vi "Designing Message Loop.vi"(8 "error in (no error)":errorcluster, 9 "Data Queue":refnum<queue>, 10 "Data Notifier":refnum<notifier>, 11 "Message Queues":T1) -> (0 "error out":errorcluster)   [LabVIEW 2025]
uses:
  support/Message Queue/All Message Queues.ctl
  support/Message Queue/Message Cluster.ctl
  controls/Tuners.ctl
  controls/Constants.ctl
  Designing Loop Enum.ctl
  <vilib>/Utility/error.llb/Error Cluster From Error Code.vi
  <vilib>/ErrorRing/Error Ring.xnode
  support/Message Queue/Message Queue.lvlib
  Results.ctl
panel:
  # "Simulator Fit"
  # "Empirical Fit"
  # "="
  # "P"
  # "* X"
  # "P"
  # "="
  # "* X"
  # "drop"
  # "drop"
  # "Simulator Fit"
  # "Empirical Fit"
  # "="
  # "P"
  # "* X"
  # "P"
  # "="
  # "* X"
  # "drop"
  # "drop"
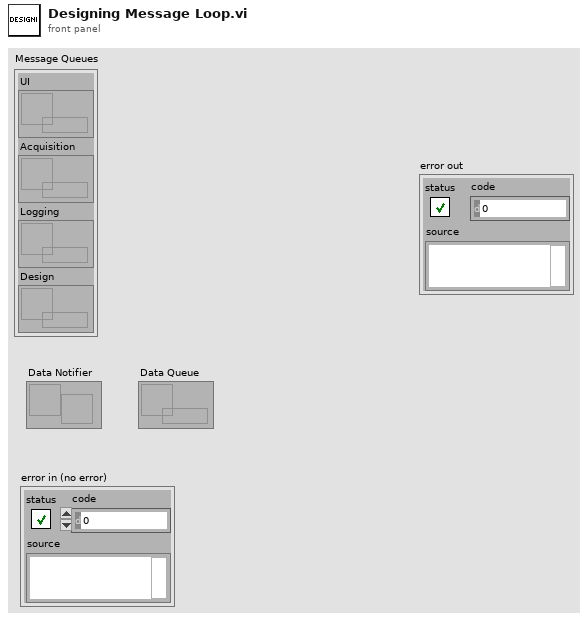
[diagram p1: front panel]
types:
  T1 = typedef "Message Queue.lvlib/All Message Queues.ctl" = cluster{"UI":refnum<queue>, "Acquisition":refnum<queue>, "Logging":refnum<queue>, "Design":refnum<queue>}
  T2 = typedef "Designing Loop Enum.ctl" = enum16{"Output New Results", "Start"}
  T3 = typedef "Results.ctl" = cluster{"Waveform":waveform(dbl), "Design Results":cluster{"Model Validation: Simulated vs. Empirical Airflow Data":cluster{dbl[], dbl[]}[], "Amplitude - Empirical":string, "Power - Empirical":string, "Amplitude - Sim":string, "Power - Sim":string, "Flow Type":u32, "Optimized Inlet \nOrifice Diameter (in)":dbl, "Flow Type Name":string}}
  T4 = typedef "Constants.ctl" = cluster{"P_amb (psia)":dbl, "T_in (Deg F)":dbl, "R_air (ft*lbf)/(lbm*R)":dbl, "g_c (lbm*ft)/(lbf*s^2)":dbl, "specific heat ratio":dbl, "Viscousity (lbm)/(ft*s)":dbl, "Cd":dbl, "Mass Flow (lbm/min) vs. Pressure Drop (inH2O) - Real Data":dbl[][]}
  T5 = typedef "Tuners.ctl" = cluster{"Inlet Diameter (in)":dbl, "Outlet Diameter (in)":dbl, " Length (in)":dbl, "   Diameter (in)":dbl, "D_h (in)":dbl, "OAR":dbl, "Run Optimizer":bool}
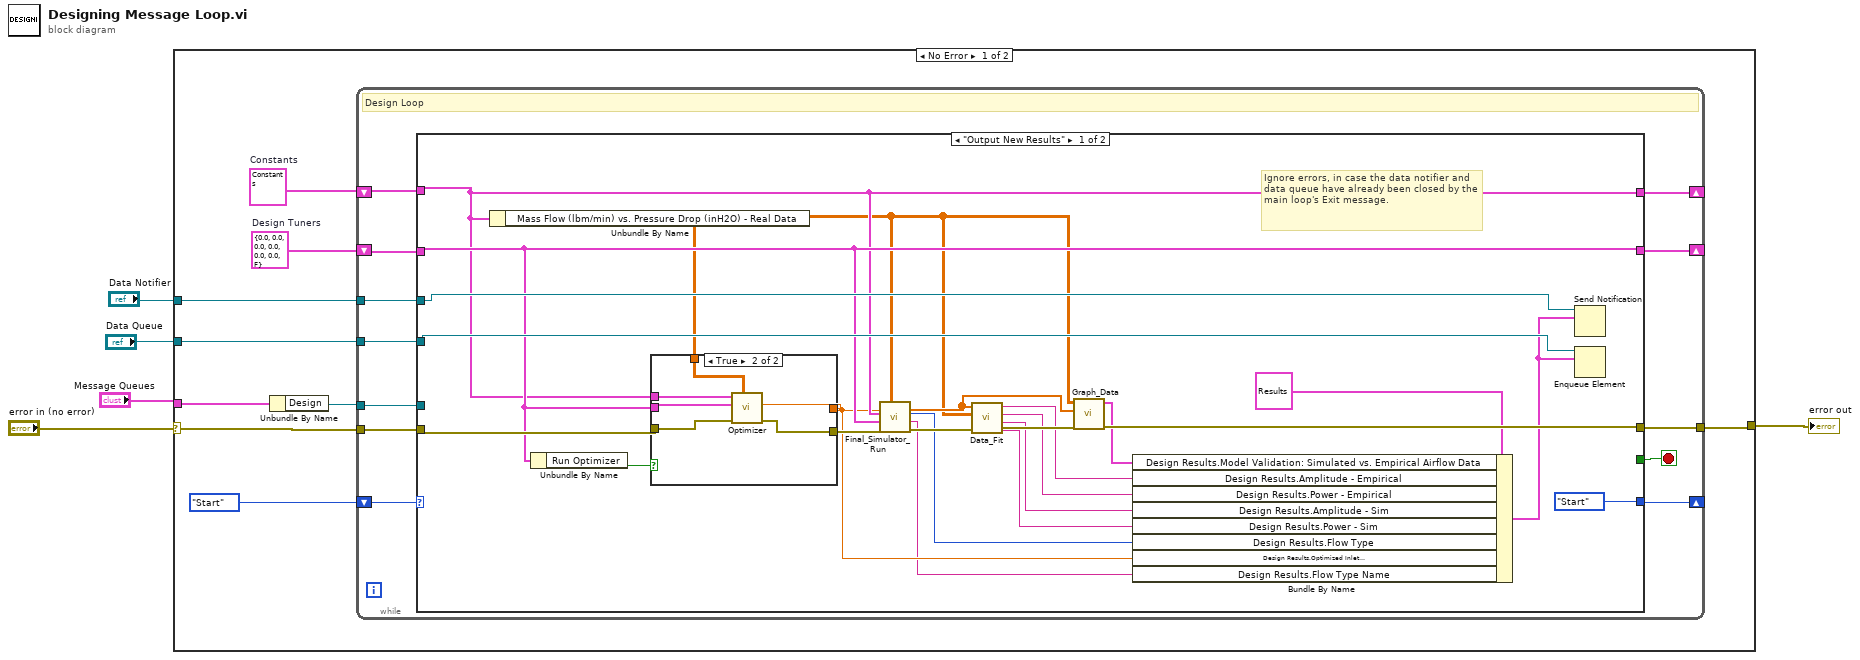
[diagram p0: block diagram]
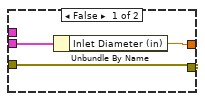
[diagram p2: hidden frame]
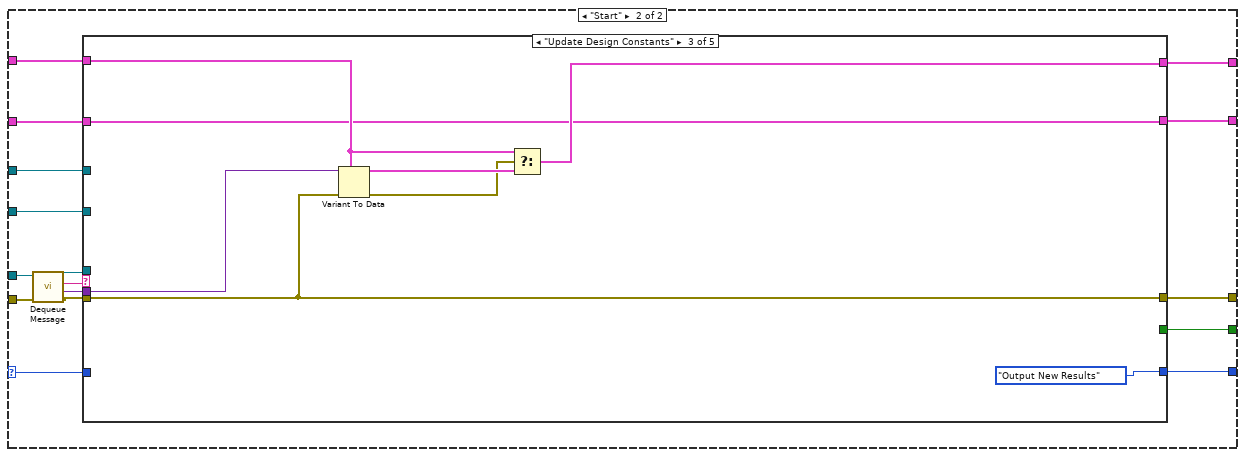
[diagram p3: hidden frame]
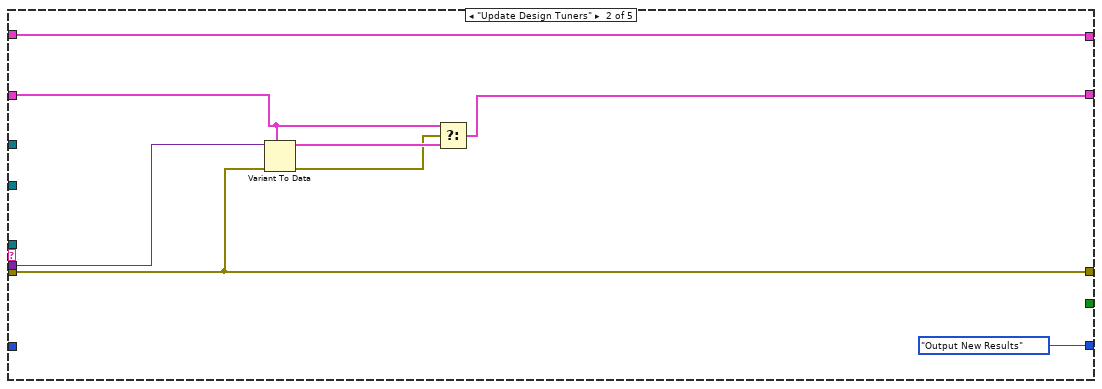
[diagram p5: hidden frame]
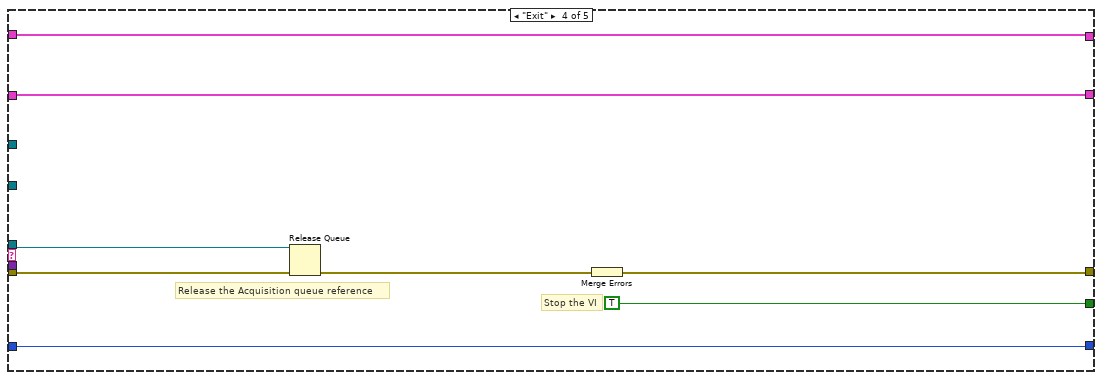
[diagram p6: hidden frame]
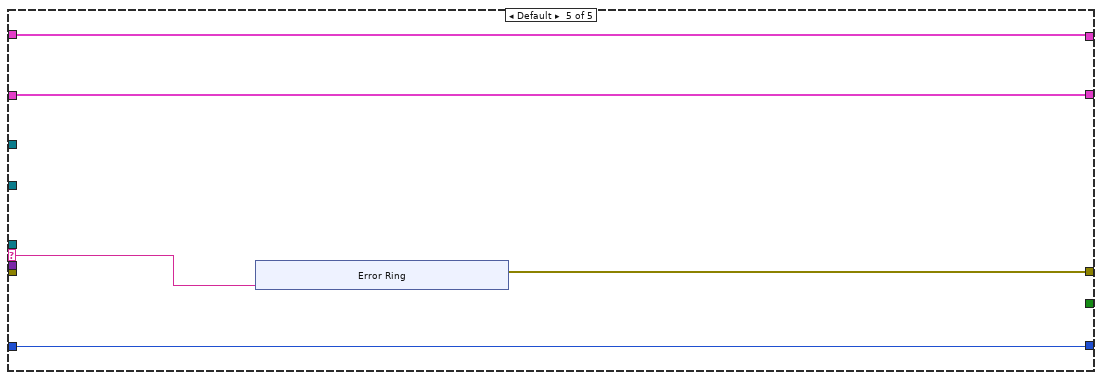
[diagram p7: hidden frame]
diagram:
  n1 = case shown="No Error" "error in (no error)" {
    selector: "error in (no error)" -> [w12 w115]
    tunnel: "Message Queues" -> [w14 _]
    tunnel: [w11 w115] -> w3
    tunnel: "Data Notifier" -> [w8 _]
    tunnel: "Data Queue" -> [w7 _]
    frame No Error {
      w9 = T4 {"P_amb (psia)"=14.7, "T_in (Deg F)"=530.0, "R_air (ft*lbf)/(lbm*R)"=53.35, "g_c (lbm*ft)/(lbf*s^2)"=32.17, "specific heat ratio"=1.4, "Viscousity (lbm)/(ft*s)"=1.21e-05, "Cd"=0.61, "Mass Flow (lbm/min) vs. Pressure Drop (inH2O) - Real Data"=[[0.5, 0.015], [1.0, 0.062], [1.5, 0.141], [2.0, 0.252], [2.5, 0.395], [3.5, 0.778]]}  # Constants
      w10 = T5 {"Inlet Diameter (in)"=0.0, "Outlet Diameter (in)"=0.0, " Length (in)"=0.0, "   Diameter (in)"=0.0, "D_h (in)"=0.0, "OAR"=0.0, "Run Optimizer"=FALSE}  # Design Tuners
      n2 = Unbundle By Name(w14) -> ("Design"=w13:refnum<queue>)
      n3 = while {
        tunnel: w13 -> [w26]
        tunnel: w12 -> [w25]
        tunnel: [w24] -> w11
        shift-right: [w22] -> _
        shift-left: w10 -> [w23]
        shift-right: [w20] -> _
        shift-left: w9 -> [w21]
        tunnel: w8 -> [w18]
        tunnel: w7 -> [w17]
        shift-right: [w15] -> _
        shift-left: Designing_Loop_Enum."Start" -> [w16]
        stop <- w19 stop-if-true
        # "Design Loop"
        n4 = case shown="\"Output New Results\"" w16 {
          selector: w16 -> [_ w59]
          tunnel: w26 -> [_ w74]
          tunnel: w25 -> [w42 w72]
          tunnel: [w41 w71] -> w24
          tunnel: w23 -> [w39 w69]
          tunnel: [w39 w68] -> w22
          tunnel: w21 -> [w38 w66]
          tunnel: [w38 w65] -> w20
          tunnel: [_ w64] -> w19
          tunnel: w18 -> [w44 w62]
          tunnel: w17 -> [w43 w61]
          tunnel: [Designing_Loop_Enum."Start" w60] -> w15
          frame "Output New Results" {
            # "Ignore errors, in case the data notifier and data queue have already been closed by the main loop's Exit message."
            n5 = Unbundle By Name(w38) -> ("Mass Flow (lbm/min) vs. Pressure Drop (inH2O) - Real Data"=w37:dbl[][])
            n6 = Unbundle By Name(w39) -> ("Run Optimizer"=w45:bool)
            n7 = case shown="True" w45 {
              tunnel: [w52 w54] -> w46
              tunnel: [w50 w58] -> w29
              tunnel: w42 -> [w52 w57]
              tunnel: w39 -> [w51 w55]
              tunnel: w37 -> [_ w56]
              tunnel: w38 -> [_ w53]
              frame False {
                n8 = Unbundle By Name(w51) -> ("Inlet Diameter (in)"=w50:dbl)
              }
              frame True {
                n9 = call "Optimizer.vi"("Mass Flow (lbm/min) vs. Pressure Drop (inH2O) - Real Data"=w56, "error in"=w57, "Tuners"=w55, "System Configuration"=w53) -> ("error out"=w54:errorcluster, "optimized_diameter"=w58:dbl)  [unwired: 6 in]
              }
            }
            n10 = call "Final_Simulator_Run.vi"("Mass Flow (lbm/min) vs. Pressure Drop (inH2O) - Real Data"=w37, "error in (no error)"=w46, "Tuners"=w39, "System Configuration"=w38, "d_in_guess"=w29) -> ("error out"=w48:errorcluster, "Flow Type Name"=w28:string, "Flow Type"=w30:u32, "total_dp_inh2o"=w47:dbl[])  [unwired: 3 in]
            n11 = call "Data_Fit.vi"("error in (no error)"=w48, "Mass Flow (lbm/min) vs. Pressure Drop (inH2O) - Real Data"=w37, "total_dp_inh2o"=w47) -> ("Power - Sim"=w31:string, "Amplitude - Sim"=w32:string, "Power - Empirical"=w33:string, "Amplitude - Empirical"=w34:string, "error out"=w49:errorcluster)  [unwired: 4 in]
            n12 = call "Graph_Data.vi"("error in (no error)"=w49, "total_dp_inh2o"=w47, "Mass Flow (lbm/min) vs. Pressure Drop (inH2O) - Real Data"=w37) -> ("error out"=w41:errorcluster, "Model Validation"=w35:cluster{dbl[], dbl[]}[])  [unwired: 7 in]
            n13 = Bundle By Name(cluster=T3 {"Waveform"={"t0"=timestamp(0 s since 1904-01-01), "dt"=1.0, "Y"=[]}, "Design Results"={"Model Validation: Simulated vs. Empirical Airflow Data"=[], "Amplitude - Empirical"="", "Power - Empirical"="", "Amplitude - Sim"="", "Power - Sim"="", "Flow Type"=0, "Optimized Inlet \nOrifice Diameter (in)"=0.0, "Flow Type Name"=""}} ("Results 2"), "Design Results.Model Validation: Simulated vs. Empirical Airflow Data"=w35, "Design Results.Amplitude - Empirical"=w34, "Design Results.Power - Empirical"=w33, "Design Results.Amplitude - Sim"=w32, "Design Results.Power - Sim"=w31, "Design Results.Flow Type"=w30, "Design Results.Optimized Inlet \nOrifice Diameter (in)"=w29, "Design Results.Flow Type Name"=w28) -> (w27:T3)
            n14 = Send Notification(notification=w27, notifier=w44) -> ()  [unwired: 1 in, 2 out]
            n15 = Enqueue Element(queue=w43, element=w27) -> ()  [unwired: 2 in, 3 out]
          }
          frame "Start" {
            n16 = call "Dequeue Message.vi"("error in (no error)"=w72, "Message Queue"=w74) -> ("error out"=w70:errorcluster, "Message Data"=w67:variant, "Message"=w73:string, "dup Message Queue"=w63:refnum<queue>)  [unwired: 6 in]
            n17 = case shown="\"Update Design Constants\"" w73 {
              selector: w73 -> [_ _ _ _ w107]
              tunnel: [w78 w83 w92 w99 w106] -> w71
              tunnel: w70 -> [w78 w83 w92 w97 _]
              tunnel: w69 -> [w77 w82 w88 w101 w104]
              tunnel: [w77 w84 w88 w101 w104] -> w68
              tunnel: w67 -> [_ w81 w91 _ _]
              tunnel: w66 -> [w76 w80 w90 w102 w105]
              tunnel: [w76 w80 w89 w102 w105] -> w65
              tunnel: [_ _ _ TRUE _] -> w64
              tunnel: w63 -> [_ _ _ w96 _]
              tunnel: w62 -> [_ _ _ _ _]
              tunnel: w61 -> [_ _ _ _ _]
              tunnel: [w75 Designing_Loop_Enum."Output New Results" Designing_Loop_Enum."Output New Results" w95 w103] -> w60
              tunnel: w59 -> [w75 _ _ w95 w103]
              frame "Initialize" {
              }
              frame "Update Design Tuners" {
                n18 = Variant To Data(error in=w83, type=w82, Variant=w81) -> (data=w86:T5, error out=w85:errorcluster)
                n19 = Select(t=w82, s=w85, f=w86) -> (s? t:f=w84:T5)
              }
              frame "Update Design Constants" {
                n20 = Variant To Data(error in=w92, type=w90, Variant=w91) -> (data=w94:T4, error out=w93:errorcluster)
                n21 = Select(t=w90, s=w93, f=w94) -> (s? t:f=w89:T4)
              }
              frame "Exit" {
                # "Release the Acquisition queue reference"
                # "Stop the VI"
                n22 = Release Queue(queue=w96, error in (no error)=w97) -> (error out=w100:errorcluster)  [unwired: 1 in, 2 out]
                n23 = Merge Errors(w100) -> (w99:errorcluster)
              }
              frame Default {
                n24 = xnode "Error Ring"("parameter 0"=w107) -> ("error out"=w106:errorcluster)
              }
            }
          }
        }
      }
    }
    frame Error {
    }
  }
  "error out" <- w3
